vi "Configure N Teeth M Missing.vi"(8 "error in (no error)":errorcluster, 10 "NTeeth Configs":T1[](array[typedef]), 11 "FPGA Interface Base in":refnum<class "FPGA Interface Base.lvclass">) -> (0 "error out":errorcluster, 3 "FPGA Interface Base out":refnum<class "FPGA Interface Base.lvclass">)   [LabVIEW 2011, in "Engine Sim RT.lvlib"]
uses:
  Engine Sim RT.lvlib
  <userlib>/_FPGA Interface Advanced Tools/FPGA Interface Base/FPGA Interface Base.lvclass
  Shared/NTeethConfig.ctl
  <userlib>/_FPGA Interface Advanced Tools/FPGA Interface Base/FPGA Write By Name - Boolean.vi
  <userlib>/_FPGA Interface Advanced Tools/FPGA Interface Base/FPGA Write By Name - U64.vi
  <userlib>/_FPGA Interface Advanced Tools/FPGA Interface Base/FPGA Write By Name - U8.vi
  Engine Simulation Shared.lvlib
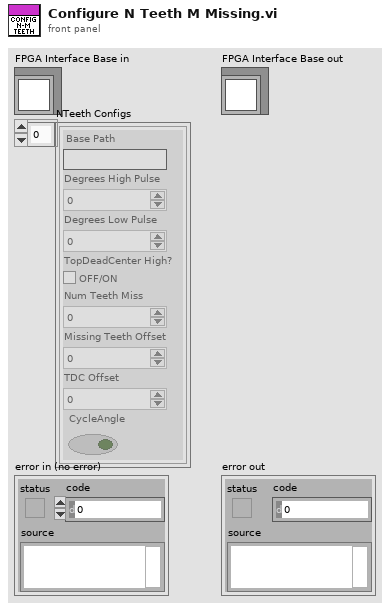
[diagram p1: front panel]
types:
  T1 = typedef "Engine Simulation Shared.lvlib/NTeethConfig.ctl" = cluster{"Base Path":string, "Degrees High Pulse":u64, "Degrees Low Pulse":u64, "TopDeadCenter High?":bool, "Num Teeth Miss":u8, "Missing Teeth Offset":u64, "TDC Offset":u64, "CycleAngle":bool}
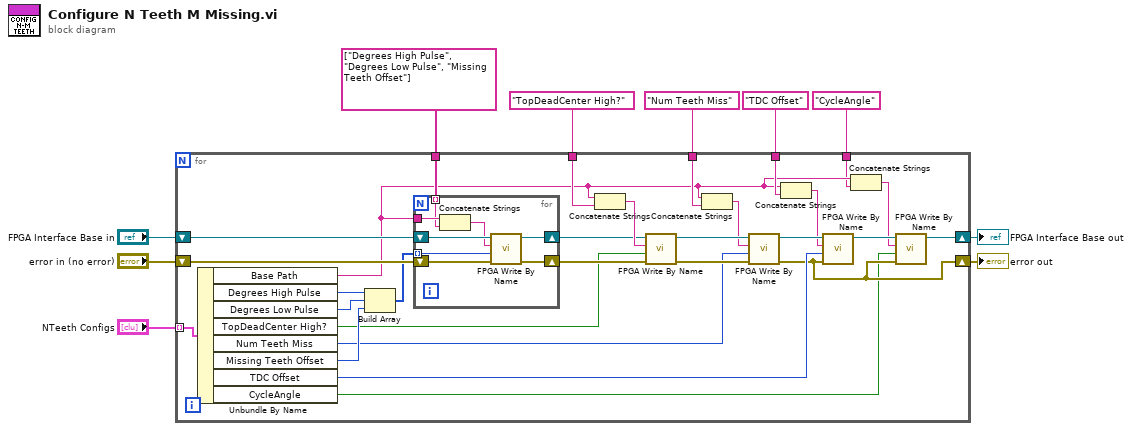
[diagram p0: block diagram]
diagram:
  n1 = for {
    shift-right: [w16] -> w5
    shift-left: "FPGA Interface Base in" -> [w33]
    shift-right: [w15] -> w6
    shift-left: "error in (no error)" -> [w35]
    tunnel: "NTeeth Configs" -> [w39] mode=indexing
    tunnel: string[] ["Degrees High Pulse", "Degrees Low Pulse", "Missing Teeth Offset"] -> [w32]
    tunnel: "TopDeadCenter High?" ("Base Path") -> [w31]
    tunnel: "Num Teeth Miss" ("Base Path") -> [w23]
    tunnel: "TDC Offset" ("Base Path") -> [w19]
    tunnel: "CycleAngle" ("Base Path") -> [w13]
    n2 = Unbundle By Name(w39) -> ("Base Path"=w14:string, "Degrees High Pulse"=w38:u64, "Degrees Low Pulse"=w37:u64, "TopDeadCenter High?"=w27:bool, "Num Teeth Miss"=w25:u8, "Missing Teeth Offset"=w36:u64, "TDC Offset"=w20:u64, "CycleAngle"=w11:bool)
    n3 = Build Array(w38, w37, w36) -> (w34:u64[])
    n4 = for {
      tunnel: w34 -> [w46] mode=indexing
      shift-right: [w41] -> w28
      shift-left: w35 -> [w47]
      shift-right: [w44] -> w29
      shift-left: w33 -> [w45]
      tunnel: w14 -> [w43]
      tunnel: w32 -> [w42] mode=indexing
      n5 = Concatenate Strings(w43, w42) -> (w40:string)
      n6 = call-poly <userlib>:"FPGA Write By Name.vi"("error in (no error)"=w47, "Value"=w46, "Control"=w40, "FPGA Session In"=w45) -> ("error out"=w41:errorcluster, "FPGA Session Out"=w44:refnum<class "FPGA Interface Base.lvclass">)  [unwired: 6 in]
    }
    n7 = Concatenate Strings(w14, w31) -> (w30:string)
    n8 = call-poly <userlib>:"FPGA Write By Name.vi"("error in (no error)"=w28, "Value"=w27, "Control"=w30, "FPGA Session In"=w29) -> ("error out"=w26:errorcluster, "FPGA Session Out"=w24:refnum<class "FPGA Interface Base.lvclass">)  [unwired: 6 in]
    n9 = Concatenate Strings(w14, w23) -> (w22:string)
    n10 = call-poly <userlib>:"FPGA Write By Name.vi"("error in (no error)"=w26, "Value"=w25, "Control"=w22, "FPGA Session In"=w24) -> ("error out"=w15:errorcluster, "FPGA Session Out"=w21:refnum<class "FPGA Interface Base.lvclass">)  [unwired: 6 in]
    n11 = Concatenate Strings(w14, w19) -> (w18:string)
    n12 = call-poly <userlib>:"FPGA Write By Name.vi"("error in (no error)"=w15, "Value"=w20, "Control"=w18, "FPGA Session In"=w21) -> ("FPGA Session Out"=w17:refnum<class "FPGA Interface Base.lvclass">)  [unwired: 6 in, 1 out]
    n13 = Concatenate Strings(w14, w13) -> (w12:string)
    n14 = call-poly <userlib>:"FPGA Write By Name.vi"("error in (no error)"=w15, "Value"=w11, "Control"=w12, "FPGA Session In"=w17) -> ("FPGA Session Out"=w16:refnum<class "FPGA Interface Base.lvclass">)  [unwired: 6 in, 1 out]
  }
  "error out" <- w6
  "FPGA Interface Base out" <- w5
